vi "Destroy SEQ.vi"(8 "error in":errorcluster, 11 "Module ID":i32) -> (0 "error out":errorcluster)   [LabVIEW 2024, in "PLC.lvlib" / "Local Instance Events SEQ.lvlib"]
doc: "_____\nCreated using DQMH Framework: Event Scripter 7.1.0.1503."
uses:
  Local Instance Events SEQ.lvlib
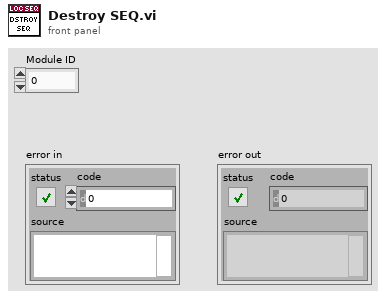
[diagram p1: front panel]
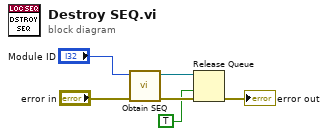
[diagram p0: block diagram]
diagram:
  n1 = call "Obtain SEQ.vi"("error in"="error in", "Module ID"="Module ID") -> ("error out"=w5:errorcluster, "Local Instance Event SEQ"=w2:refnum<queue>)  [unwired: 7 in, 1 out]
  n2 = Release Queue(queue=w2, force destroy? (F)=TRUE, error in (no error)=w5) -> (error out=→"error out":errorcluster)  [unwired: 2 out]
